vi "Get Type Name.vi"(11 "DMM in":refnum<class "DMM.lvclass">) -> (2 "Type Name":string)   [LabVIEW 2020, in "2. Basic Panel Actors.lvlib" / "DMM.lvclass"]
doc: "Returns the instrument type name.\n----\nCopyright: MGI 2017\nAuthor: Derek Trepanier"
uses:
  DMM.lvclass
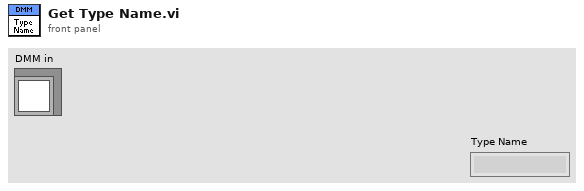
[diagram p1: front panel]
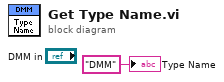
[diagram p0: block diagram]
diagram:
  "Type Name" <- "DMM" ("Type Name")
